vi "Read Result Data.vi"(0 "VISA resource name":refnum<visa-resource-name>, 5 "Result Number (1-200) (1)":i32=1 min=1 max=8, 11 "error in (no error)":errorcluster) -> (4 "VISA resource name out":refnum<visa-resource-name>, 6 "Test Data Cluster":T2, 15 "error out":errorcluster)   [LabVIEW 2016, in "eec EST 300.lvlib"]
doc: "RD n? Where n is the desired step number.\n\nRetrieves the parsed data step result from the previously run test. Note you will not get a result until after the step has completed."
uses:
  <instrlib>/eec EST 300/eec EST 300.lvlib
  <instrlib>/eec EST 300/Public/Configure/Steps/Low Level/Test Type.ctl
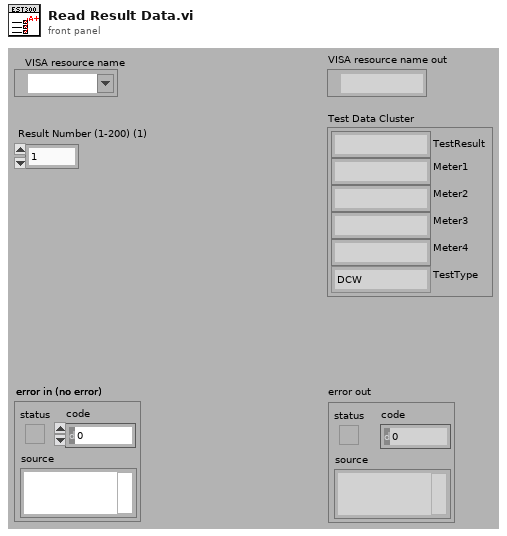
[diagram p1: front panel]
types:
  T1 = typedef "eec EST 300.lvlib/Test Type.ctl" = enum16{"DCW", "IR", "ACW"}
  T2 = cluster{"TestResult":string, "Meter1":string, "Meter2":string, "Meter3":string, "Meter4":string, "TestType":T1}
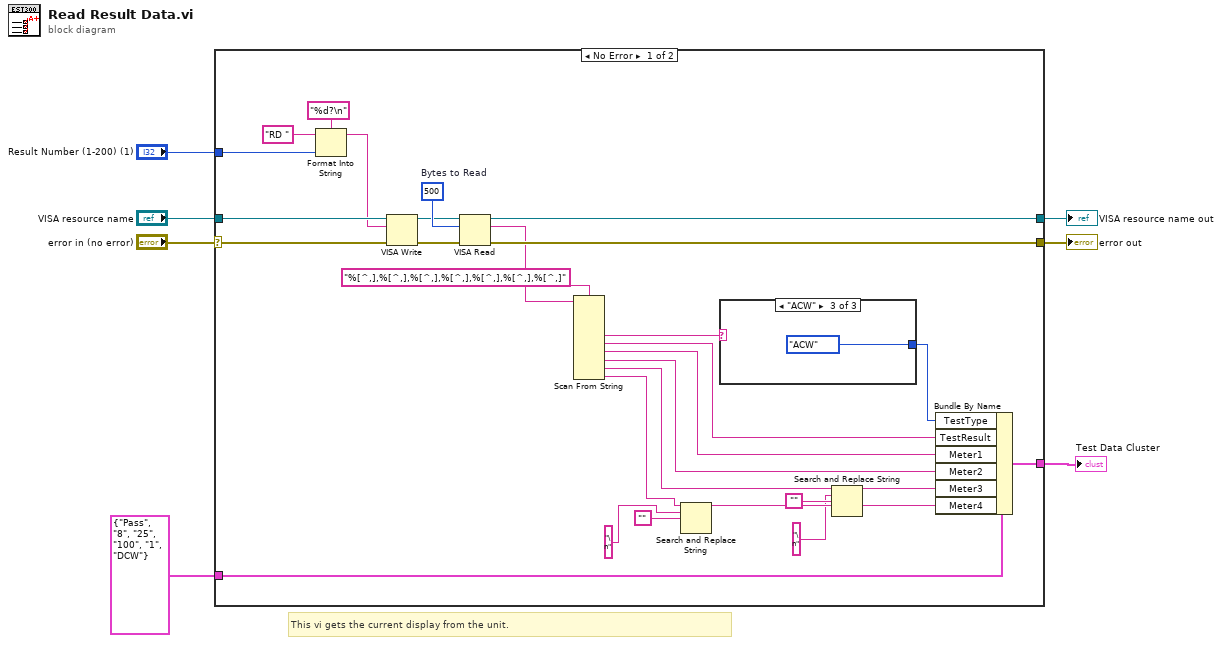
[diagram p0: block diagram]
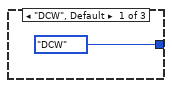
[diagram p2: hidden frame]
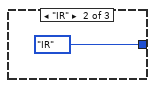
[diagram p3: hidden frame]
diagram:
  # "This vi gets the current display from the unit."
  n1 = case shown="No Error" "error in (no error)" {
    selector: "error in (no error)" -> [w35 w41]
    tunnel: [w32 w41] -> w6
    tunnel: [w31 w40] -> w4
    tunnel: "VISA resource name" -> [w34 w40]
    tunnel: "Result Number (1-200) (1)" -> [w33 _]
    tunnel: T2 {"TestResult"="Pass", "Meter1"="8", "Meter2"="25", "Meter3"="100", "Meter4"="1", "TestType"=enum."DCW"} ("Test Data Cluster") -> [w29 w39]
    tunnel: [w28 w39] -> w2
    frame No Error {
      w24 = u32 500  # Bytes to Read
      n2 = Format Into String(format string="%d?\n", initial string="RD " ("string (\"\")"), w33) -> (resulting string=w25:string)  [unwired: 1 in, 1 out]
      n3 = VISA Write(VISA resource name=w34, write buffer=w25, error in (no error)=w35) -> (VISA resource name out=w22:refnum<visa-resource-name>, error out=w23:errorcluster)  [unwired: 1 out]
      n4 = VISA Read(VISA resource name=w22, byte count=w24, error in (no error)=w23) -> (VISA resource name out=w31:refnum<visa-resource-name>, read buffer=w30:string, error out=w32:errorcluster)  [unwired: 1 out]
      n5 = Scan From String(format string="%[^,],%[^,],%[^,],%[^,],%[^,],%[^,],%[^,]", input string=w30) -> (output 2=w17:string, output 3=w18:string, output 4=w19:string, output 5=w20:string, output 6=w11:string, output 7=w14:string)  [unwired: 10 in, 3 out]
      n6 = Search and Replace String(input string=w14, search string="\n", replace string="") -> (result string=w13:string)  [unwired: 5 in, 3 out]
      n7 = case shown="\"ACW\"" w17 {
        tunnel: [Test_Type."DCW" ("TestType") Test_Type."IR" ("TestType") Test_Type."ACW" ("TestType")] -> w16
        frame "DCW", Default {
        }
        frame "IR" {
        }
        frame "ACW" {
        }
      }
      n8 = Search and Replace String(input string=w11, search string="\n", replace string="") -> (result string=w10:string)  [unwired: 5 in, 3 out]
      n9 = Bundle By Name(cluster=w29, "TestType"=w16, "TestResult"=w18, "Meter1"=w19, "Meter2"=w20, "Meter3"=w10, "Meter4"=w13) -> (w28:T2)
    }
    frame Error {
    }
  }
  "error out" <- w6
  "VISA resource name out" <- w4
  "Test Data Cluster" <- w2
